vi "Identify.vi"(8 "error in (no error)":errorcluster, 11 "Config Parser BML in":refnum<class "Config Parser BML.lvclass">) -> (0 "error out":errorcluster, 2 "Plugin is Valid":bool, 3 "Config Parser BML out":refnum<class "Config Parser BML.lvclass">)   [LabVIEW 2018, in "Config Parser BML.lvlib" / "Config Parser BML.lvclass"]
uses:
  Config Parser BML.lvclass
  C:/P4 Workspace/PC Client/Solutions/5g_eap/trunk/1.0/HiSi5GmmWave/Pattern_Gen_Tool/Interfaces/File Parser Interface.lvlibp/Interfaces/File Parser Interface/File Parser Interface.lvclass
  Interfaces/File Parser Interface.lvlibp/Ctls/Protocol Type.ctl
  Interfaces/File Parser Interface.lvlibp/Interfaces/File Parser Interface/Read Protocol Type.vi
  Interfaces/File Parser Interface.lvlibp
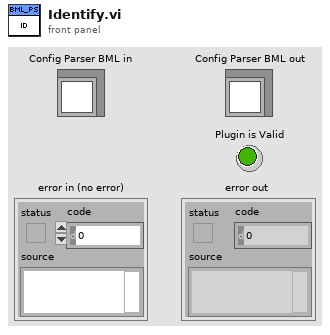
[diagram p1: front panel]
types:
  T1 = typedef "File Parser Interface.lvlibp/Protocol Type.ctl" = enum16{"BML_LS", "BML_HS", "SPI_3W", "SPI_4W"}
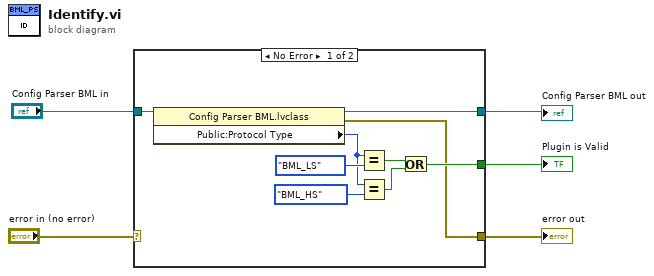
[diagram p0: block diagram]
diagram:
  n1 = case shown="No Error" "error in (no error)" {
    selector: "error in (no error)" -> [_ w15]
    tunnel: "Config Parser BML in" -> [w14 w16]
    tunnel: [w8 _] -> w3
    tunnel: [w7 w15] -> w2
    tunnel: [w6 w16] -> w1
    frame No Error {
      n2 = property class="Config Parser BML.lvclass"(reference=w14) -> (reference out=w6:refnum<class "Config Parser BML.lvclass">, error out=w7:errorcluster, "Public:Protocol Type"=w12:T1)  [unwired: 1 in]
      n3 = Equal?(x=w12, y=Protocol_Type."BML_LS") -> (x = y?=w9:bool)
      n4 = Equal?(x=w12, y=Protocol_Type."BML_HS") -> (x = y?=w10:bool)
      n5 = Or(x=w9, y=w10) -> (x .or. y?=w8:bool)
    }
    frame Error {
    }
  }
  "error out" <- w2
  "Config Parser BML out" <- w1
  "Plugin is Valid" <- w3
